vi "FlatToRichni_measurementlink_discovery_v1_EnumerateServicesResponse.vi"(5 "OutputClusterType":T1, 11 "InputCluster":T4) -> (3 "OutputCluster":T1)   [LabVIEW 2020, in "Measurement Plugin Discovery Client.lvlib"]
uses:
  Measurement Plugin Discovery Client.lvlib
  ni_measurementlink_discovery_v1_EnumerateServicesResponse_Flat.ctl
  ni_measurementlink_discovery_v1_ServiceDescriptor_Flat.ctl
  ni_measurementlink_discovery_v1_ServiceDescriptor_AnnotationsEntry_Flat.ctl
  ni_measurementlink_discovery_v1_EnumerateServicesResponse.ctl
  ni_measurementlink_discovery_v1_ServiceDescriptor.ctl
  ni_measurementlink_discovery_v1_ServiceDescriptor_AnnotationsEntry.ctl
  FlatToRichni_measurementlink_discovery_v1_ServiceDescriptor_AnnotationsEntry.vi
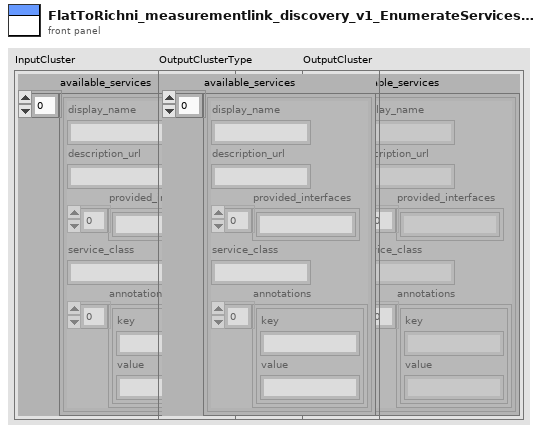
[diagram p1: front panel]
types:
  T1 = typedef "Measurement Plugin Discovery Client.lvlib/ni_measurementlink_discovery_v1_EnumerateServicesResponse.ctl" = cluster{"available_services":T2[]}
  T2 = typedef "Measurement Plugin Discovery Client.lvlib/ni_measurementlink_discovery_v1_ServiceDescriptor.ctl" = cluster{"display_name":string, "description_url":string, "provided_interfaces":string[], "service_class":string, "annotations":T3[]}
  T3 = typedef "Measurement Plugin Discovery Client.lvlib/ni_measurementlink_discovery_v1_ServiceDescriptor_AnnotationsEntry.ctl" = cluster{"key":string, "value":string}
  T4 = typedef "Measurement Plugin Discovery Client.lvlib/ni_measurementlink_discovery_v1_EnumerateServicesResponse_Flat.ctl" = cluster{"available_services":T5[]}
  T5 = typedef "Measurement Plugin Discovery Client.lvlib/ni_measurementlink_discovery_v1_ServiceDescriptor_Flat.ctl" = cluster{"display_name":string, "description_url":string, "provided_interfaces":string[], "service_class":string, "annotations":T6[]}
  T6 = typedef "Measurement Plugin Discovery Client.lvlib/ni_measurementlink_discovery_v1_ServiceDescriptor_AnnotationsEntry_Flat.ctl" = cluster{"key":string, "value":string}
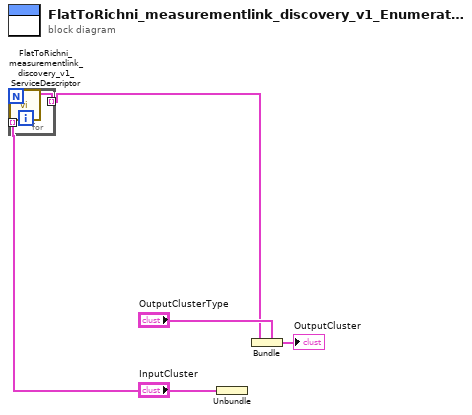
[diagram p0: block diagram]
diagram:
  n1 = Unbundle "Unbundle"("InputCluster") -> ("available_services"=w2:T5[])
  n2 = for {
    tunnel: w2 -> [w7] mode=indexing
    tunnel: [w6] -> w1 mode=indexing
    n3 = call "FlatToRichni_measurementlink_discovery_v1_ServiceDescriptor.vi"("InputCluster"=w7) -> ("OutputCluster"=w6:T2)  [unwired: 10 in]
  }
  n4 = Bundle "Bundle"(cluster="OutputClusterType", "available_services"=w1) -> (→"OutputCluster":T1)
